vi "Generate Traffic on CAN Bus.vi"() -> ()   [LabVIEW 2025]
uses:
  <resource>/objmgr/xnet.rc
  <vilib>/xnet/xnet.llb/XNET Frame Type CAN.ctl
  <vilib>/xnet/xnet.llb/XNET Frame CAN.ctl
  <vilib>/xnet/xnet.llb/XNET Create Session (Frame Output Stream).vi
  <vilib>/numeric/Random Number (Range) U64.vi
  <vilib>/xnet/xnet.llb/XNET Write (Frame CAN).vi
panel:
  in  "Select Interface":refnum<k21>="CAN2"
  out "Gen error out":errorcluster
  in  "Generate":bool
  in  "stop":bool
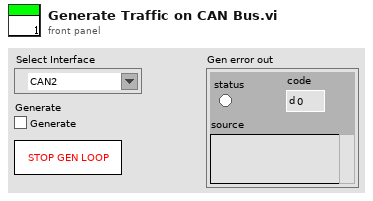
[diagram p1: front panel]
types:
  T1 = typedef "XNET Frame CAN.ctl" = cluster{"timestamp":timestamp, "payload":u8[], "identifier":u32, "type":T2, "extended?":bool, "echo?":bool}
  T2 = typedef "XNET Frame Type CAN.ctl" = u8
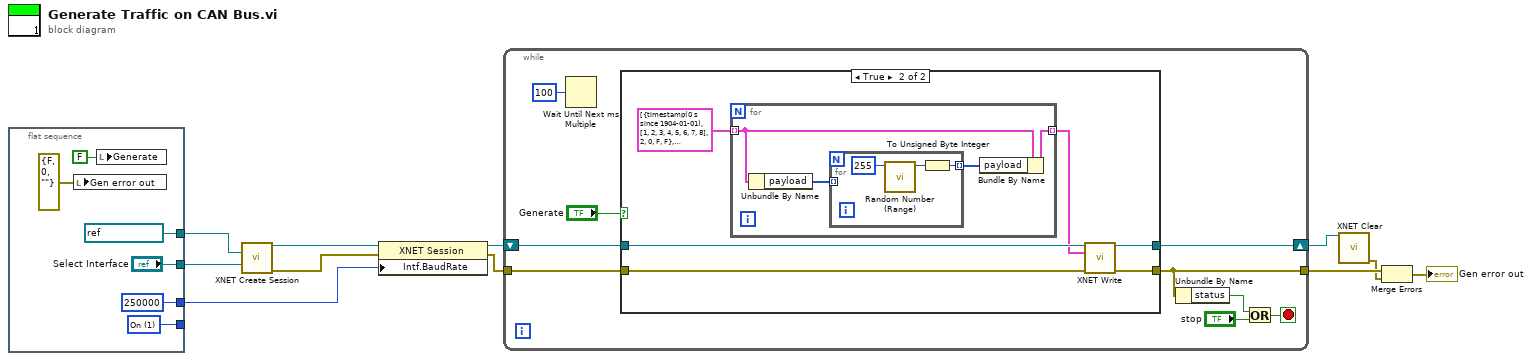
[diagram p0: block diagram]
diagram:
  n1 = flat-sequence {
    tunnel: ["Select Interface"] -> w11
    tunnel: [u32 250000 ("Interface Baud Rate")] -> w8
    tunnel: [refnum<k21> ":memory:" ("CAN Cluster")] -> w5
    tunnel: [w12] -> _
    frame #0 {
      w12 = u32 1 items=["Off", "On"] ("Interface:CAN:Termination")
      n2 = local write "Gen error out"(errorcluster {"status"=FALSE, "code"=0, "source"=""} ("Gen error out")) -> ()
      n3 = local write "Generate"(FALSE ("Generate")) -> ()
    }
  }
  n4 = call-poly <vilib>:"XNET Create Session.vi"("cluster (:memory:)"=w5, "interface"=w11) -> ("session out"=w10:refnum<k21>, "error out"=w6:errorcluster)  [unwired: 1 in, 11 out]
  n5 = property class="XNET Session"(reference=w10, error in=w6, "Intf.BaudRate"=w8) -> (reference out=w9:refnum<k21>, error out=w7:errorcluster)
  n6 = while {
    tunnel: w7 -> [w24]
    tunnel: [w23] -> w4
    shift-right: [w18] -> w3
    shift-left: w9 -> [w25]
    stop <- w19 stop-if-true
    n7 = Wait Until Next ms Multiple(millisecond multiple=u32 100 ("milliseconds to wait")) -> ()  [unwired: 1 out]
    n8 = case shown="True" "Generate" {
      tunnel: w25 -> [w27 w34]
      tunnel: w24 -> [w28 w33]
      tunnel: [w28 w32] -> w23
      tunnel: [w27 w29] -> w18
      frame False {
      }
      frame True {
        n9 = for {
          tunnel: [w36] -> w30 mode=indexing
          tunnel: T1[] [{"timestamp"=timestamp(0 s since 1904-01-01), "payload"=[1, 2, 3, 4, 5, 6, 7, 8], "identifier"=2, "type"=0, "extended?"=FALSE, "echo?"=FALSE}, {"timestamp"=timestamp(0 s since 1904-01-01), "payload"=[0, 1, 2, 3, 4, 5, 6, 7], "identifier"=3, "type"=0, "extended?"=FALSE, "echo?"=FALSE}] ("data") -> [w38] mode=indexing
          n10 = Unbundle By Name(w38) -> ("payload"=w37:u8[])
          n11 = for {
            tunnel: w37 -> [_] mode=indexing
            tunnel: [w39] -> w35 mode=indexing
            n12 = call-poly <vilib>:"Random Number (Range).vi"("upper bound (100)"=u64 255) -> ("number"=w40:u64)  [unwired: 10 in]
            n13 = To Unsigned Byte Integer(number=w40) -> (unsigned 8bit integer=w39:u8)
          }
          n14 = Bundle By Name(cluster=w38, "payload"=w35) -> (w36:T1)
        }
        n15 = call-poly <vilib>:"XNET Write.vi"("session in"=w34, "data"=w30, "error in (no error)"=w33) -> ("session out"=w29:refnum<k21>, "error out"=w32:errorcluster)  [unwired: 11 out]
      }
    }
    n16 = Unbundle By Name(w23) -> ("status"=w26:bool)
    n17 = Or(x=w26, y="stop") -> (x .or. y?=w19:bool)
  }
  n18 = call <vilib>:"XNET Clear.vi"("session in"=w3) -> ("error out"=w1:errorcluster)  [unwired: 14 in]
  n19 = Merge Errors(w4, w1) -> (→"Gen error out":errorcluster)
